vi "V002 - Variable DC Controller - Auto Controlling Without Buttons.vi"() -> ()   [LabVIEW 2022 SP3]
uses:
  <vilib>/DAQmx/read.llb/DAQmx Read (Analog DBL 1Chan 1Samp).vi
  <vilib>/DAQmx/create/channels.llb/DAQmx Create Channel (AI-Voltage-Basic).vi
  <vilib>/DAQmx/miscellaneous.llb/DAQmx Fill In Error Info.vi
panel:
  out "Case 1 reached":bool
  out "CH2 Appl":bool
  in  "Appl CH2":bool
  out "Power On 3":bool
  out "Power On 2":bool
  in  "Turn On CH3":bool
  in  "Turn On CH2":bool
  out "Case 2  Reached":bool
  out "Case 1 Reached":bool
  in  "Numeric Controller Sub":dbl format="%#_1g"
  out "Power On":bool
  in  "Turn On CH1":bool
  out "Case 0 Reached":bool
  out "Connected":bool
  in  "VISA resource name":refnum<visa-resource-name>
  in  "Connect":bool
  in  "Numeric Controller Main":dbl
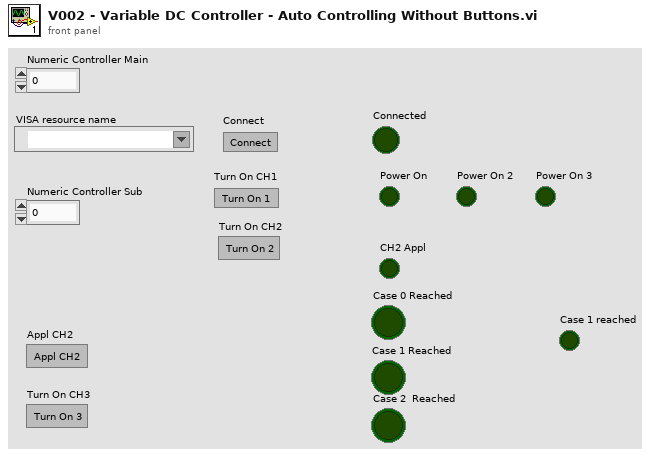
[diagram p1: front panel]
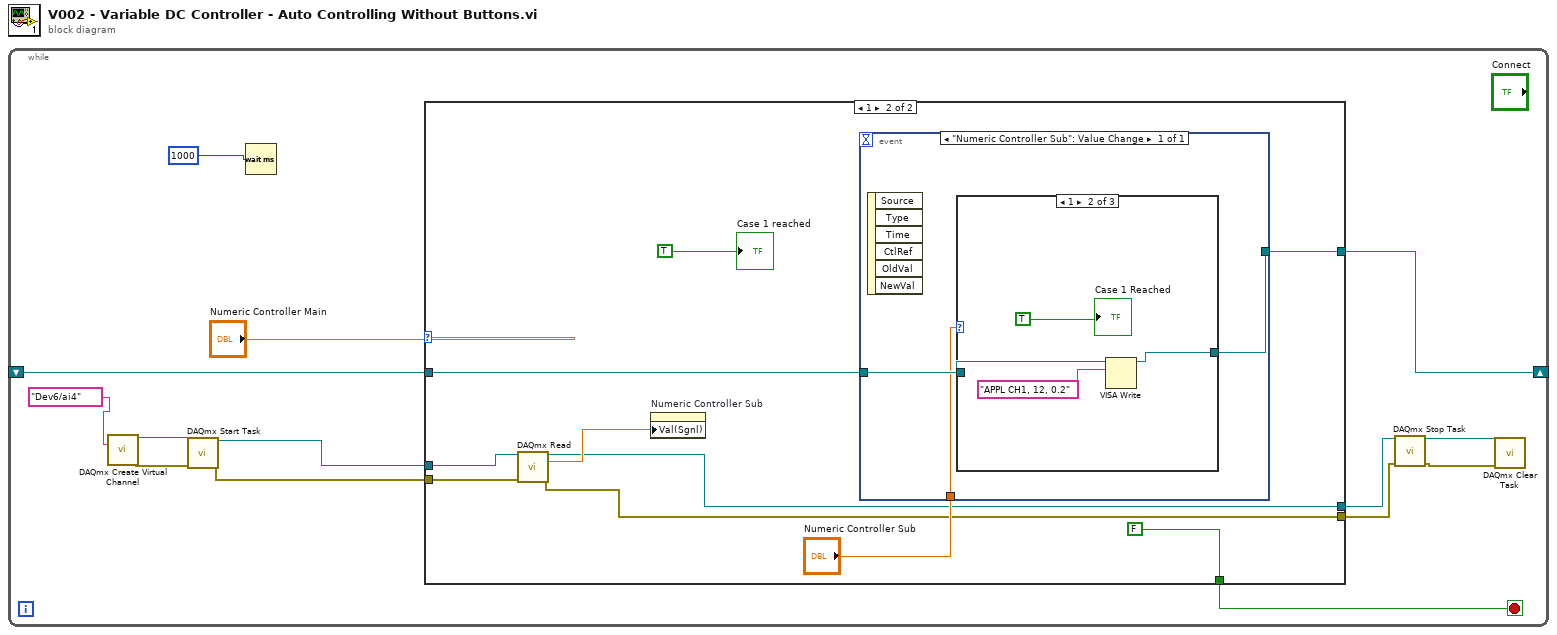
[diagram p0: block diagram]
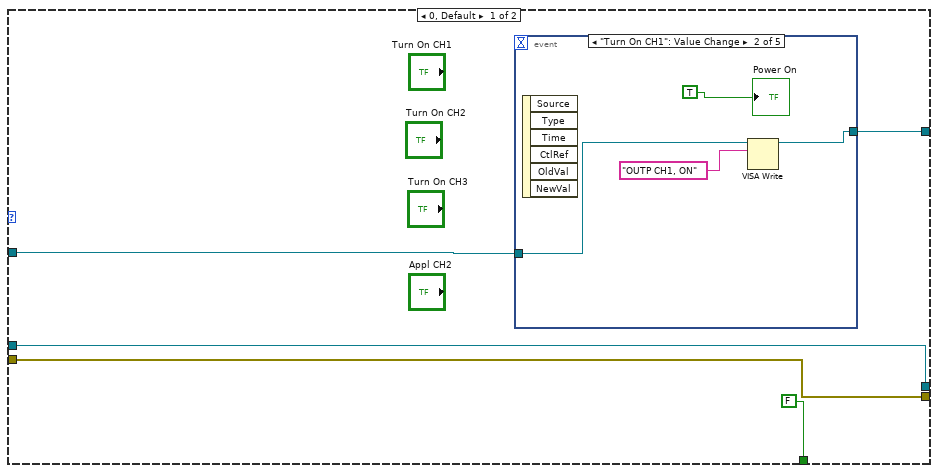
[diagram p2: hidden frame]
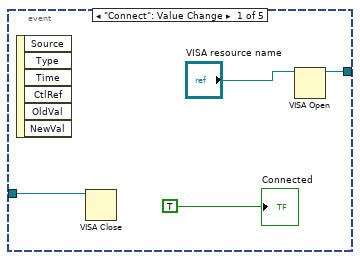
[diagram p3: hidden frame]
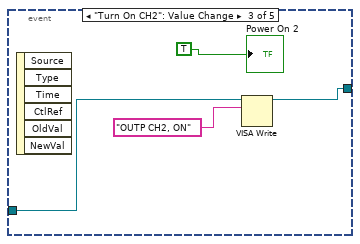
[diagram p4: hidden frame]
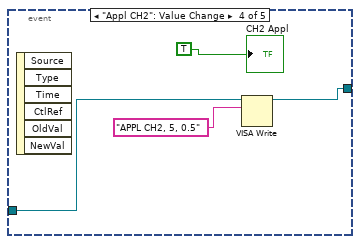
[diagram p5: hidden frame]
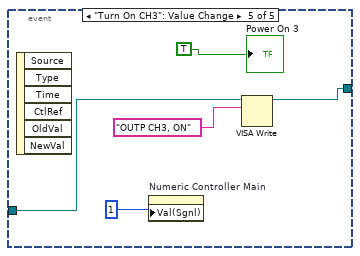
[diagram p6: hidden frame]
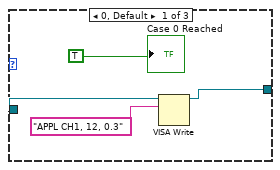
[diagram p7: hidden frame]
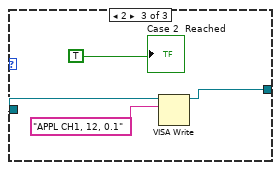
[diagram p8: hidden frame]
diagram:
  n1 = while {
    shift-right: [w13] -> _
    shift-left: _ -> [w14]
    stop <- w12 stop-if-true
    n2 = call-poly <vilib>:"DAQmx Create Virtual Channel.vi"("physical channels"=tag "Dev6/ai4") -> ("task out"=w10:refnum<k21>, "error out"=w6:errorcluster)  [unwired: 13 in]
    n3 = call <vilib>:"DAQmx Start Task.vi"("task/channels in"=w10, "error in"=w6) -> ("task out"=w8:refnum<k21>, "error out"=w7:errorcluster)  [unwired: 12 in]
    n4 = Wait (ms)(milliseconds to wait=1000) -> ()  [unwired: 1 out]
    n5 = case shown="1" "Numeric Controller Main" {
      tunnel: w14 -> [w19 w48]
      tunnel: [w18 w49] -> w13
      tunnel: [FALSE FALSE] -> w12
      tunnel: w8 -> [w16 w45]
      tunnel: w7 -> [w15 w43]
      tunnel: [w16 w42] -> w2
      tunnel: [w15 w41] -> w1
      frame 0, Default {
        n6 = event shown="[1] \"Turn On CH1\": Value Change" {
          selector: _ -> [_ _ _ _ _]
          dyn-events: _ -> [_ _ _ _ _]
          timeout: _ -> [_ _ _ _ _]
          tunnel: w19 -> [w23 w26 w30 w34 w39]
          tunnel: [w22 w25 w29 w33 w38] -> w18
          event "Connect": Value Change {
            n7 = event-data() -> ()  [unwired: 1 in, 6 out]
            n8 = VISA Close(VISA resource name=w23) -> ()  [unwired: 1 in, 1 out]
            n9 = VISA Open(VISA resource name="VISA resource name") -> (VISA resource name=w22:refnum<visa-resource-name>)  [unwired: 4 in, 1 out]
            "Connected" <- TRUE
          }
          event "Turn On CH1": Value Change {
            n10 = event-data() -> ()  [unwired: 1 in, 6 out]
            n11 = VISA Write(VISA resource name=w26, write buffer="OUTP CH1, ON") -> (VISA resource name out=w25:refnum<visa-resource-name>)  [unwired: 1 in, 2 out]
            "Power On" <- TRUE
          }
          event "Turn On CH2": Value Change {
            n12 = event-data() -> ()  [unwired: 1 in, 6 out]
            n13 = VISA Write(VISA resource name=w30, write buffer="OUTP CH2, ON") -> (VISA resource name out=w29:refnum<visa-resource-name>)  [unwired: 1 in, 2 out]
            "Power On 2" <- TRUE
          }
          event "Appl CH2": Value Change {
            n14 = event-data() -> ()  [unwired: 1 in, 6 out]
            n15 = VISA Write(VISA resource name=w34, write buffer="APPL CH2, 5, 0.5") -> (VISA resource name out=w33:refnum<visa-resource-name>)  [unwired: 1 in, 2 out]
            "CH2 Appl" <- TRUE
          }
          event "Turn On CH3": Value Change {
            n16 = event-data() -> ()  [unwired: 1 in, 6 out]
            n17 = property on="Numeric Controller Main" class="DigNum (strict)"("Val(Sgnl)"=1) -> ()  [unwired: 2 in, 2 out]
            n18 = VISA Write(VISA resource name=w39, write buffer="OUTP CH3, ON") -> (VISA resource name out=w38:refnum<visa-resource-name>)  [unwired: 1 in, 2 out]
            "Power On 3" <- TRUE
          }
        }
      }
      frame 1 {
        n19 = call-poly <vilib>:"DAQmx Read.vi"("task/channels in"=w45, "error in"=w43) -> ("task out"=w42:refnum<k21>, "data"=w46:dbl, "error out"=w41:errorcluster)  [unwired: 11 in]
        n20 = property on="Numeric Controller Sub" class="DigNum (strict)"("Val(Sgnl)"=w46) -> ()  [unwired: 2 in, 2 out]
        n21 = event shown="[0] \"Numeric Controller Sub\": Value Change" {
          selector: _ -> [_]
          dyn-events: _ -> [_]
          timeout: _ -> [_]
          tunnel: [w53] -> w49
          tunnel: w48 -> [w52]
          tunnel: "Numeric Controller Sub" -> [w51]
          event "Numeric Controller Sub": Value Change {
            n22 = event-data() -> ()  [unwired: 1 in, 6 out]
            n23 = case shown="1" w51 {
              tunnel: [w56 w60 w64] -> w53
              tunnel: w52 -> [w55 w59 w63]
              frame 0, Default {
                n24 = VISA Write(VISA resource name=w55, write buffer="APPL CH1, 12, 0.3") -> (VISA resource name out=w56:refnum<visa-resource-name>)  [unwired: 1 in, 2 out]
                "Case 0 Reached" <- TRUE
              }
              frame 1 {
                n25 = VISA Write(VISA resource name=w59, write buffer="APPL CH1, 12, 0.2") -> (VISA resource name out=w60:refnum<visa-resource-name>)  [unwired: 1 in, 2 out]
                "Case 1 Reached" <- TRUE
              }
              frame 2 {
                n26 = VISA Write(VISA resource name=w63, write buffer="APPL CH1, 12, 0.1") -> (VISA resource name out=w64:refnum<visa-resource-name>)  [unwired: 1 in, 2 out]
                "Case 2  Reached" <- TRUE
              }
            }
          }
        }
        "Case 1 reached" <- TRUE
      }
    }
    n27 = call <vilib>:"DAQmx Stop Task.vi"("task/channels in"=w2, "error in"=w1) -> ("task out"=w4:refnum<k21>, "error out"=w3:errorcluster)  [unwired: 12 in]
    n28 = call <vilib>:"DAQmx Clear Task.vi"("task in"=w4, "error in"=w3) -> ()  [unwired: 13 in, 1 out]
  }
